vi "getFilesPathByDialog.vi"(8 "error in (no error)":errorcluster) -> (0 "error out":errorcluster, 2 "pathLvlibDir":path, 3 "pathIdl":path)   [LabVIEW 2018]
doc: "Get the idl and lvlib file paths by dialog."
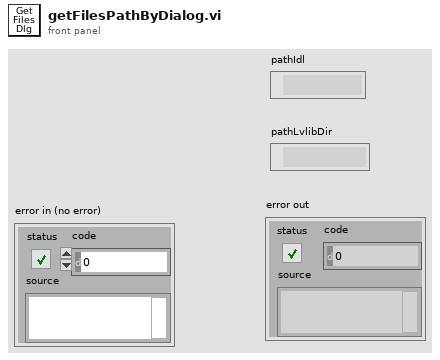
[diagram p1: front panel]
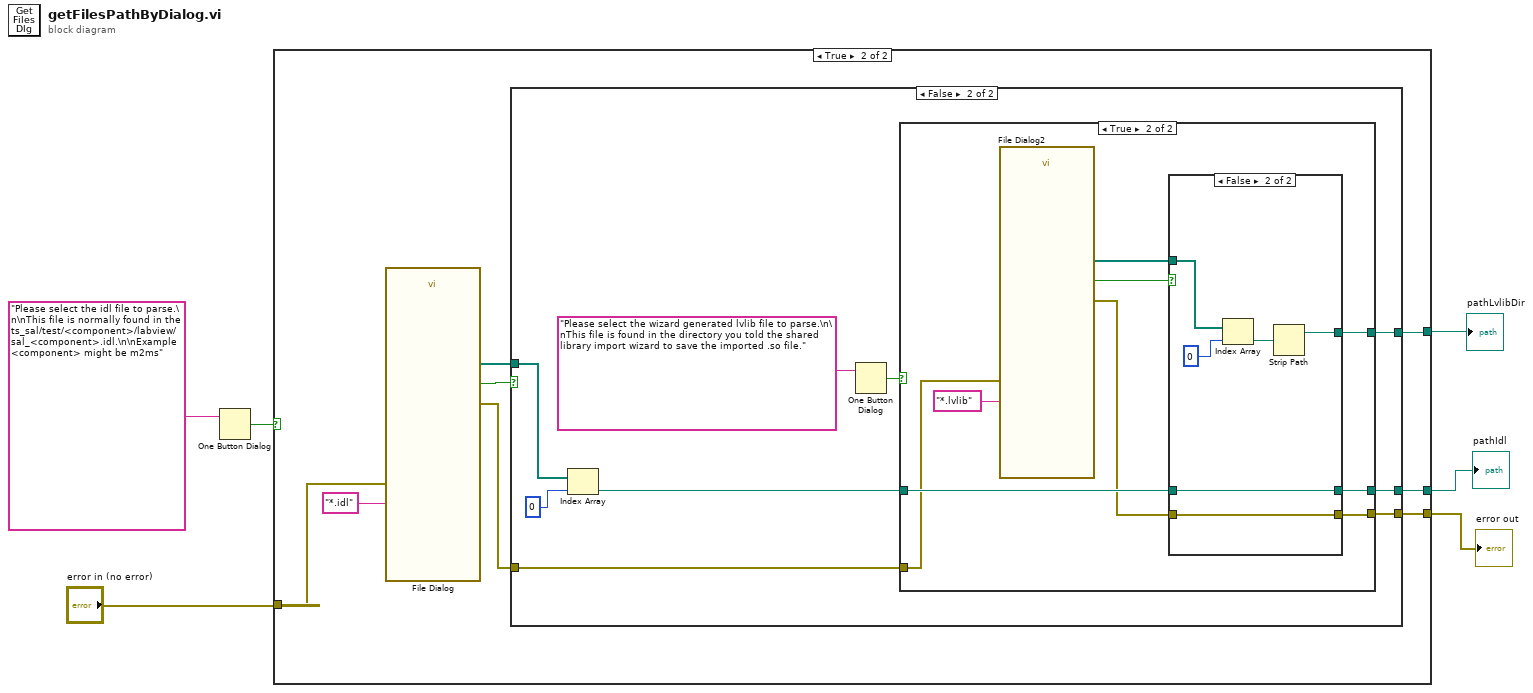
[diagram p0: block diagram]
diagram:
  n1 = One Button Dialog(message="Please select the idl file to parse.\n\nThis file is normally found in the ts_sal/test/<component>/labview/sal_<component>.idl.\n\nExample <component> might be m2ms") -> (true=w5:bool)  [unwired: 1 in]
  n2 = case shown="True" w5 {
    tunnel: [w7 w13] -> w3
    tunnel: "error in (no error)" -> [w7 w8]
    tunnel: [_ w11] -> w2
    tunnel: [_ w10] -> w1
    frame False {
    }
    frame True {
      n3 = call "File Dialog"("error in"=w8, "pattern (all files)"="*.idl") -> ("selected paths"=w15:path[], "cancelled"=w14:bool, "error out"=w9:errorcluster)  [unwired: 10 in, 1 out]
      n4 = case shown="False" w14 {
        tunnel: w15 -> [_ w24]
        tunnel: [w16 w20] -> w13
        tunnel: w9 -> [w16 w19]
        tunnel: [_ w18] -> w11
        tunnel: [_ w17] -> w10
        frame True {
        }
        frame False {
          n5 = Index Array(array=w24, index=0) -> (element=w25:path)
          n6 = One Button Dialog(message="Please select the wizard generated lvlib file to parse.\n\nThis file is found in the directory you told the shared library import wizard to save the imported .so file.") -> (true=w21:bool)  [unwired: 1 in]
          n7 = case shown="True" w21 {
            tunnel: w25 -> [w26 w34]
            tunnel: [w27 w32] -> w20
            tunnel: w19 -> [w27 w29]
            tunnel: [_ w31] -> w18
            tunnel: [w26 w30] -> w17
            frame False {
            }
            frame True {
              n8 = call "File Dialog2"("error in"=w29, "pattern (all files)"="*.lvlib") -> ("selected paths"=w35:path[], "cancelled"=w33:bool, "error out"=w28:errorcluster)  [unwired: 10 in, 1 out]
              n9 = case shown="False" w33 {
                tunnel: w35 -> [_ w43]
                tunnel: w34 -> [w37 w39]
                tunnel: [w38 w40] -> w32
                tunnel: w28 -> [w38 w40]
                tunnel: [_ w41] -> w31
                tunnel: [w37 w39] -> w30
                frame True {
                }
                frame False {
                  n10 = Index Array(array=w43, index=0) -> (element=w42:path)
                  n11 = Strip Path(path=w42) -> (stripped path=w41:path)  [unwired: 1 out]
                }
              }
            }
          }
        }
      }
    }
  }
  "error out" <- w3
  "pathIdl" <- w1
  "pathLvlibDir" <- w2
